vi "GrabBkDataString.vi"(0 "error out 2":errorcluster, 1 "VISA resource name out 2":refnum<visa-resource-name>) -> (2 "error out":errorcluster, 3 "String":string, 4 "VISA resource name out":refnum<visa-resource-name>)   [LabVIEW 2010]
uses:
  <instrlib>/BK Precision 85XX Series/BK Precision 85XX Series.lvlib
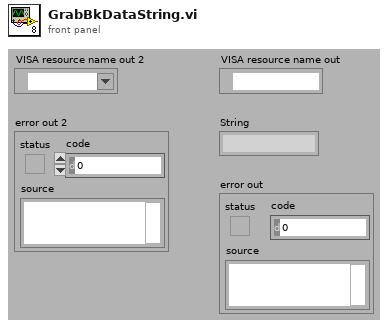
[diagram p1: front panel]
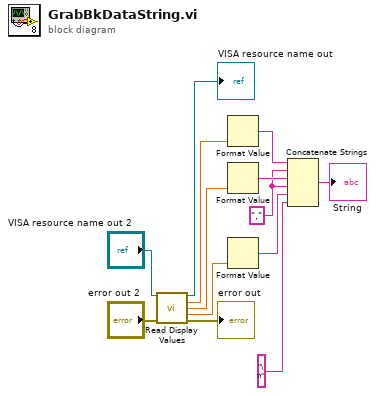
[diagram p0: block diagram]
diagram:
  w5 = ","
  n1 = call <instrlib>:"Read Display Values.vi"("VISA resource name"="VISA resource name out 2", "error in (no error)"="error out 2") -> ("VISA resource name out"=→"VISA resource name out":refnum<visa-resource-name>, "Terminal Input Voltage (V)"=w11:dbl, "Terminal Input Current (A)"=w12:dbl, "Terminal Input Power (W)"=w10:dbl, "error out"=→"error out":errorcluster)  [unwired: 9 in]
  n2 = Format Value(value (0)=w11) -> (output string=w9:string)  [unwired: 2 in]
  n3 = Format Value(value (0)=w12) -> (output string=w8:string)  [unwired: 2 in]
  n4 = Format Value(value (0)=w10) -> (output string=w7:string)  [unwired: 2 in]
  n5 = Concatenate Strings(w9, w5, w8, w5, w7, "\n") -> (→"String":string)
